vi "Setting Window.vi"(11 "GUI.lvlib:GUI.lvclass":refnum<class "GUI.lvclass">) -> ()   [LabVIEW 2020, in "GUI.lvlib" / "GUI.lvclass"]
uses:
  GUI.lvclass
  GUI.lvclass/GUI.ctl
panel:
  in  "Period":u16 caption="Период опроса, мс"
  in  "OK Button":bool
  in  "Close Button":bool
  in  "Stand LAI slave":u16 caption="Стенд. LAI"
  in  "Stand LDO slave":u16 caption="Стенд. LDO"
  in  "Control module slave":u16 caption="Проверяемый модуль"
  in  "Parity":bool caption="Контроль четности"
  in  "Скорость обмена, бод":u16(ring)=9600 items=["1200"=1200, "2400"=2400, "9600"=9600]
  # "Настройки"
  # "Modbus. Slave-адреса"
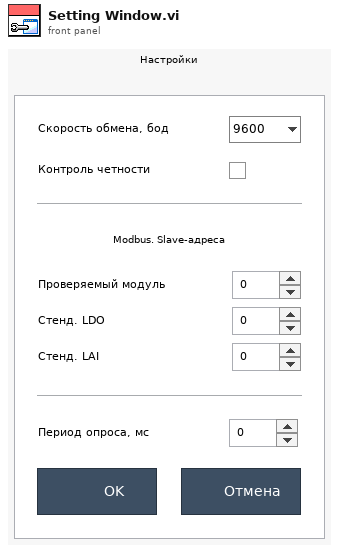
[diagram p1: front panel]
types:
  T1 = enum32{"Invalid", "Standard", "Closed", "Hidden", "Minimized", "Maximized"}
  T2 = typedef "Port Settings.ctl" = cluster{"VISA resource":string, "BAUD":u16, "Parity":bool, "LDO":u16, "LAI":u16, "Control":u16, "Period":u16}
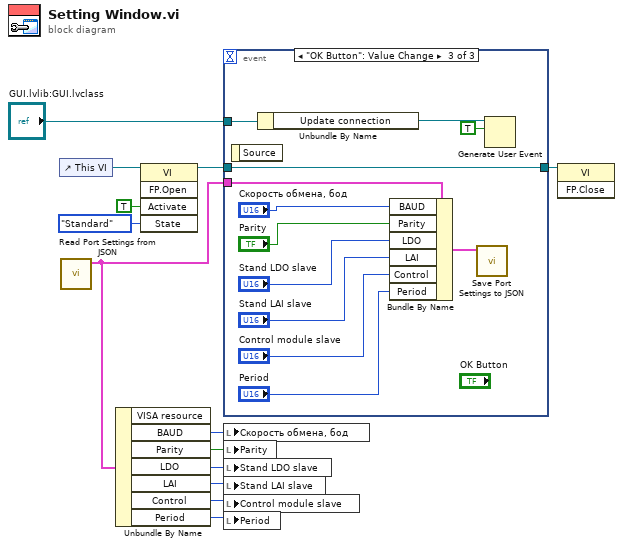
[diagram p0: block diagram]
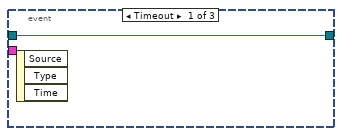
[diagram p2: hidden frame]
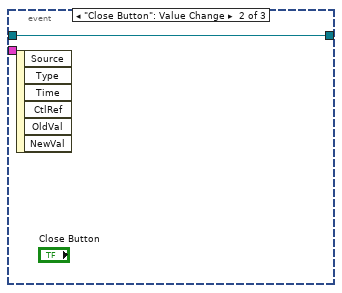
[diagram p3: hidden frame]
diagram:
  n1 = control-ref of="This VI"() -> (w13:refnum<vi>)
  n2 = call "Read Port Settings from JSON.vi"() -> ("Port settings"=w2:T2)  [unwired: 11 in]
  n3 = Unbundle By Name(w2) -> ("BAUD"=w8:u16, "Parity"=w7:bool, "LDO"=w6:u16, "LAI"=w5:u16, "Control"=w4:u16, "Period"=w3:u16)  [unwired: 1 out]
  n4 = invoke class="VI" method="FP.Open"(reference=w13, "Activate"=TRUE ("Activate?"), "State"=T1."Standard") -> (reference out=w12:refnum<vi>)  [unwired: 2 in, 4 out]
  n5 = event shown="[2] \"OK Button\": Value Change" {
    selector: _ -> [_ _ _]
    dyn-events: _ -> [_ _ _]
    timeout: _ -> [_ _ _]
    tunnel: [w14 w15 w27] -> w9
    tunnel: w12 -> [w14 w15 w27]
    tunnel: w2 -> [_ _ w26]
    tunnel: "GUI.lvlib:GUI.lvclass" -> [_ _ w18]
    event Timeout {
      n6 = event-data() -> ()  [unwired: 1 in, 3 out]
    }
    event "Close Button": Value Change {
      n7 = event-data() -> ()  [unwired: 1 in, 6 out]
    }
    event "OK Button": Value Change {
      n8 = event-data() -> ()  [unwired: 1 in, 1 out]
      n9 = Unbundle By Name(w18) -> ("Update connection"=w17:refnum<user-event>)
      n10 = Bundle By Name(cluster=w26, "BAUD"="Скорость обмена, бод", "Parity"="Parity", "LDO"="Stand LDO slave", "LAI"="Stand LAI slave", "Control"="Control module slave", "Period"="Period") -> (w19:T2)
      n11 = call "Save Port Settings to JSON.vi"("Port settings"=w19) -> ()  [unwired: 11 in]
      n12 = Generate User Event(user event=w17, event data cluster=TRUE ("event data")) -> ()  [unwired: 2 in, 2 out]
    }
  }
  n13 = local write "Скорость обмена, бод"(w8) -> ()
  n14 = local write "Parity"(w7) -> ()
  n15 = local write "Stand LDO slave"(w6) -> ()
  n16 = local write "Stand LAI slave"(w5) -> ()
  n17 = local write "Control module slave"(w4) -> ()
  n18 = local write "Period"(w3) -> ()
  n19 = invoke class="VI" method="FP.Close"(reference=w9) -> ()  [unwired: 2 in, 3 out]
